vi "extract ROIS.vi"(8 "error in (no error)":errorcluster, 11 "Cascade in":refnum<class "Cascade.lvclass">) -> (0 "error out":errorcluster, 3 "Cascade out":refnum<class "Cascade.lvclass">)   [LabVIEW 2012, in "Cascade.lvclass"]
uses:
  Cascade.lvclass
  Cascade.lvclass/Cascade.ctl
  <vilib>/vision/NI_Vision_Development_Module.lvlib
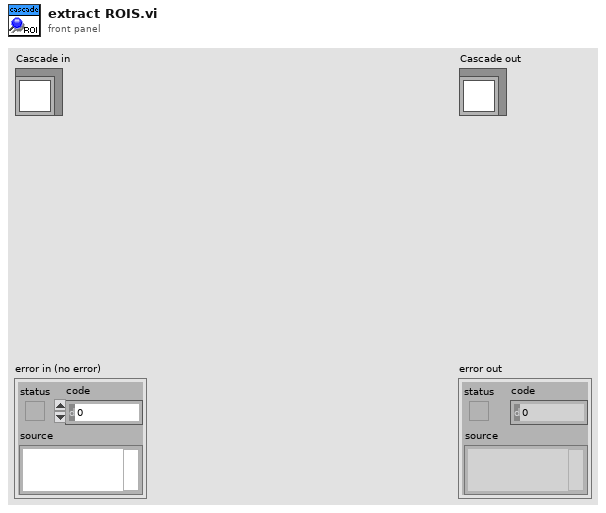
[diagram p1: front panel]
types:
  T1 = typedef "IMAQ Image.ctl" = refnum<image>
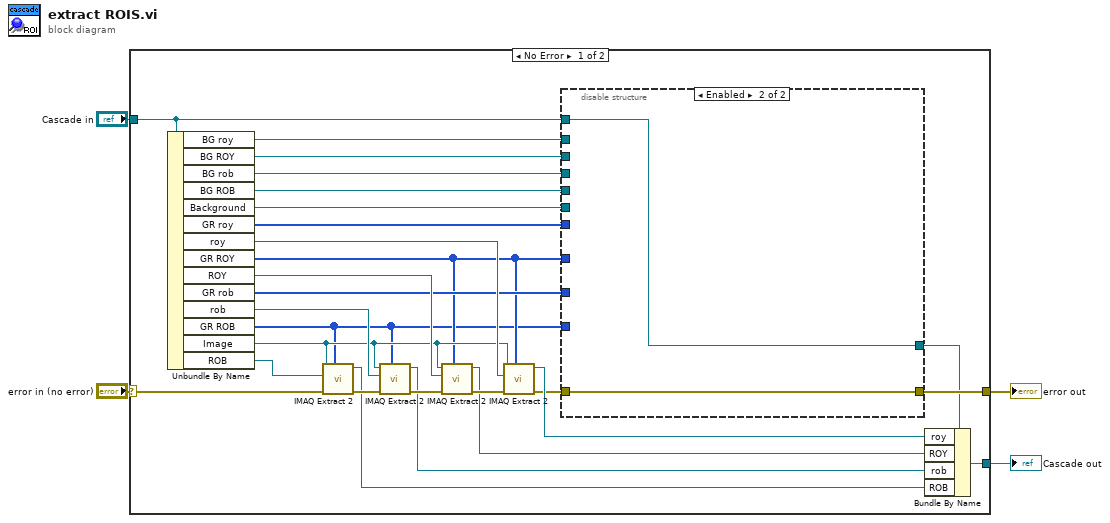
[diagram p0: block diagram]
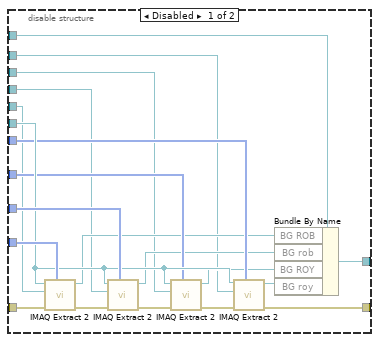
[diagram p2: hidden frame]
diagram:
  n1 = case shown="No Error" "error in (no error)" {
    selector: "error in (no error)" -> [w28 w55]
    tunnel: [w17 w55] -> w3
    tunnel: [w23 w54] -> w1
    tunnel: "Cascade in" -> [w11 w54]
    frame No Error {
      n2 = Unbundle By Name(w11) -> ("BG roy"=w7:T1, "BG ROY"=w8:T1, "BG rob"=w9:T1, "BG ROB"=w12:T1, "Background"=w14:T1, "GR roy"=w13:i32[], "roy"=w24:T1, "GR ROY"=w6:i32[], "ROY"=w25:T1, "GR rob"=w15:i32[], "rob"=w26:T1, "GR ROB"=w5:i32[], "Image"=w16:T1, "ROB"=w27:T1)
      n3 = call "IMAQ Extract 2"("Optional Rectangle"=w5, "error in (no error)"=w28, "Image Dst"=w27, "Image Src"=w16) -> ("error out"=w30:errorcluster, "Image Dst Out"=w22:T1)  [unwired: 6 in]
      n4 = call "IMAQ Extract 2"("Optional Rectangle"=w5, "error in (no error)"=w30, "Image Dst"=w26, "Image Src"=w16) -> ("error out"=w31:errorcluster, "Image Dst Out"=w21:T1)  [unwired: 6 in]
      n5 = call "IMAQ Extract 2"("Optional Rectangle"=w6, "error in (no error)"=w31, "Image Dst"=w25, "Image Src"=w16) -> ("error out"=w29:errorcluster, "Image Dst Out"=w20:T1)  [unwired: 6 in]
      n6 = call "IMAQ Extract 2"("Optional Rectangle"=w6, "error in (no error)"=w29, "Image Dst"=w24, "Image Src"=w16) -> ("error out"=w18:errorcluster, "Image Dst Out"=w19:T1)  [unwired: 6 in]
      n7 = disable-structure shown="Enabled" {
        disable-tunnel: w18 -> [w51 w53]
        disable-tunnel: [w47 w53] -> w17
        disable-tunnel: w5 -> [w46 _]
        disable-tunnel: w15 -> [w45 _]
        disable-tunnel: w14 -> [w44 _]
        disable-tunnel: w6 -> [w43 _]
        disable-tunnel: w13 -> [w42 _]
        disable-tunnel: w12 -> [w41 _]
        disable-tunnel: w11 -> [w40 w52]
        disable-tunnel: [w39 w52] -> w10
        disable-tunnel: w9 -> [w37 _]
        disable-tunnel: w8 -> [w35 _]
        disable-tunnel: w7 -> [w32 _]
        frame Disabled {
          n8 = call "IMAQ Extract 2"("Optional Rectangle"=w46, "error in (no error)"=w51, "Image Dst"=w41, "Image Src"=w44) -> ("error out"=w50:errorcluster, "Image Dst Out"=w38:T1)  [unwired: 6 in]
          n9 = call "IMAQ Extract 2"("Optional Rectangle"=w45, "error in (no error)"=w50, "Image Dst"=w37, "Image Src"=w44) -> ("error out"=w49:errorcluster, "Image Dst Out"=w36:T1)  [unwired: 6 in]
          n10 = call "IMAQ Extract 2"("Optional Rectangle"=w43, "error in (no error)"=w49, "Image Dst"=w35, "Image Src"=w44) -> ("error out"=w48:errorcluster, "Image Dst Out"=w34:T1)  [unwired: 6 in]
          n11 = call "IMAQ Extract 2"("Optional Rectangle"=w42, "error in (no error)"=w48, "Image Dst"=w32, "Image Src"=w44) -> ("error out"=w47:errorcluster, "Image Dst Out"=w33:T1)  [unwired: 6 in]
          n12 = Bundle By Name(cluster=w40, "BG ROB"=w38, "BG rob"=w36, "BG ROY"=w34, "BG roy"=w33) -> (w39:refnum<class "Cascade.lvclass">)
        }
        frame Enabled {
        }
      }
      n13 = Bundle By Name(cluster=w10, "roy"=w19, "ROY"=w20, "rob"=w21, "ROB"=w22) -> (w23:refnum<class "Cascade.lvclass">)
    }
    frame Error {
    }
  }
  "error out" <- w3
  "Cascade out" <- w1
